vi "QNET_Signal_Generator.vi"(2 "time (s)":dbl, 3 "Signal Generator Parameters":T1={"Amplitude"=2.0, "Frequency"=0.4, "Offset"=0.0, "Signal Type"=0, "Disturbance"=FALSE} {"Offset" min=-5 max=5 step=0.5 format="%#.2f"; "Frequency" min=0 step=0.1 format="%#.2f"; "Amplitude" min=0 step=0.5 format="%#.2f"}) -> (0 "Output":dbl)   [LabVIEW 2010]
doc: "Generates a square wave or sawtooth wave with a specified amplitude, frequency, and offset."
uses:
  <vilib>/ptbypt/NI_PtbyPt.lvlib
panel:
  # "V"
  # "Hz"
  # "V"
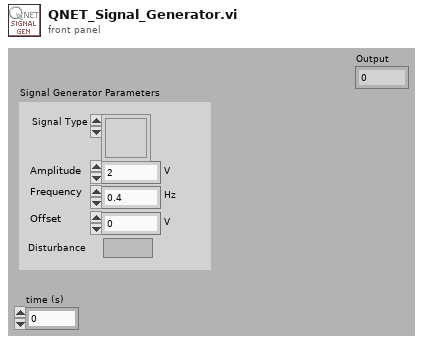
[diagram p1: front panel]
types:
  T1 = cluster{"Amplitude":sgl, "Frequency":sgl, "Offset":sgl, "Signal Type":u16, "Disturbance":bool}
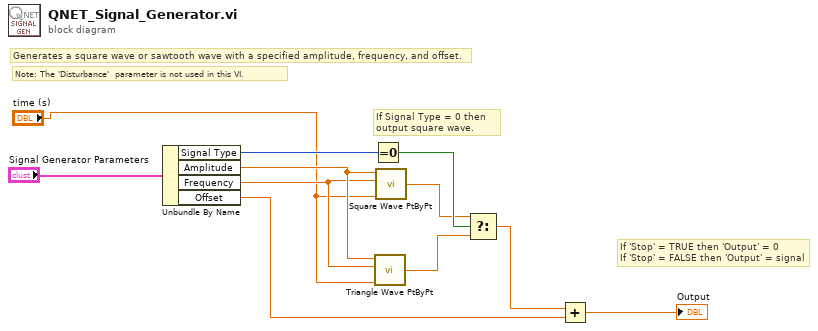
[diagram p0: block diagram]
diagram:
  # "Note: The 'Disturbance'  parameter is not used in this VI."
  # "Generates a square wave or sawtooth wave with a specified amplitude, frequency, and offset."
  # "If Signal Type = 0 then output square wave."
  # "If 'Stop' = TRUE then 'Output' = 0\nIf 'Stop' = FALSE then 'Output' = signal"
  n1 = Unbundle By Name("Signal Generator Parameters") -> ("Signal Type"=w3:u16, "Amplitude"=w6:sgl, "Frequency"=w5:sgl, "Offset"=w4:sgl)
  n2 = Equal To 0?(x=w3) -> (x = 0?=w10:bool)
  n3 = call <vilib>:"Triangle Wave PtByPt.vi"("time"="time (s)", "frequency"=w5, "amplitude"=w6) -> ("triangle wave"=w8:dbl)  [unwired: 1 in]
  n4 = call <vilib>:"Square Wave PtByPt.vi"("amplitude"=w6, "frequency"=w5, "time"="time (s)") -> ("square wave"=w9:dbl)  [unwired: 2 in]
  n5 = Select(t=w9, s=w10, f=w8) -> (s? t:f=w11:dbl)
  n6 = Add(x=w11, y=w4) -> (x+y=→"Output":dbl)
